vi "AutoDriveStraight.vi"(8 "error in (no error)":errorcluster, 9 "TimeOut (s)":dbl, 10 "MaxSpeed (ft/s)":dbl, 11 "Dist (ft)":dbl) -> (0 "error out":errorcluster)   [LabVIEW 2020]
doc: "Wrapper class for drive straight"
uses:
  <vilib>/Utility/semaphor.llb/Obtain Semaphore Reference.vi
  <vilib>/Rock Robotics/WPI/ThirdParty/JAS_Junk/TrajLib/Timer_Reset.vi
  <vilib>/Rock Robotics/WPI/ThirdParty/JAS_Junk/TrajLib/Trajectory_Library.lvlib
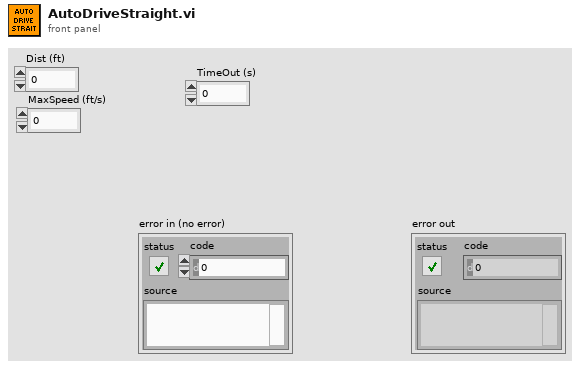
[diagram p1: front panel]
types:
  T1 = typedef "Trajectory_Library.lvlib/TIMER.ctl" = cluster{"StartTime":dbl, "Accumulated TIme":dbl, "Running":bool, "semaphore":T2}
  T2 = typedef "Semaphore RefNum" = refnum<k1>
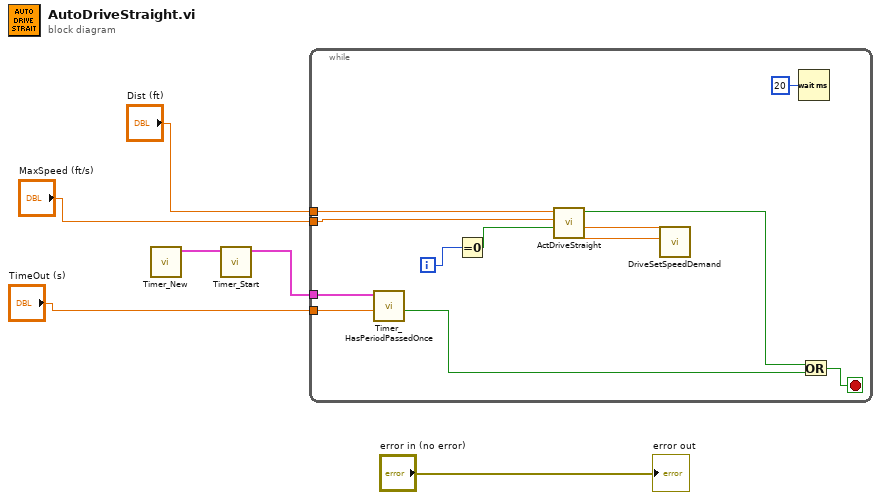
[diagram p0: block diagram]
diagram:
  n1 = call <vilib>:"Timer_New.vi"() -> ("TIMER"=w3:T1)  [unwired: 11 in]
  n2 = call <vilib>:"Timer_Start.vi"("in Timer"=w3) -> ("out Timer"=w2:T1)  [unwired: 10 in]
  n3 = while {
    tunnel: "Dist (ft)" -> [w18]
    tunnel: "MaxSpeed (ft/s)" -> [w17]
    tunnel: w2 -> [w14]
    tunnel: "TimeOut (s)" -> [w13]
    i -> [w15]
    stop <- w11 stop-if-true
    n4 = call <vilib>:"Timer_HasPeriodPassedOnce.vi"("Period"=w13, "in Timer"=w14) -> ("Expired"=w12:bool)  [unwired: 7 in, 2 out]
    n5 = Equal To 0?(x=w15) -> (x = 0?=w16:bool)
    n6 = call "ActDriveStraight.vi"("FirstTime"=w16, "MaxSpeed (ft/s)"=w17, "Dist (ft)"=w18) -> ("RightSpeedDemand"=w7:dbl, "LeftSpeedDemand"=w8:dbl, "Done"=w10:bool)  [unwired: 6 in]
    n7 = call "DriveSetSpeedDemand.vi"("RSpeedDemand (ft/s)"=w7, "LSpeedDemand (ft/s)"=w8) -> ()  [unwired: 10 in]
    n8 = Wait (ms)(milliseconds to wait=u32 20) -> ()  [unwired: 1 out]
    n9 = Or(x=w10, y=w12) -> (x .or. y?=w11:bool)
  }
  "error out" <- "error in (no error)"
